vi "Compensator.vi"() -> ()   [LabVIEW 2010]
uses:
  <vilib>/Platform/TimedLoop/XDataNode/XDataNode.xnode
  <vilib>/Platform/TimedLoop/XDataNode/timing_clust.ctl
  <vilib>/Platform/TimedLoop/XDataNode/nitl_modes.ctl
  <vilib>/Platform/TimedLoop/XDataNode/wakeup.ctl
  <vilib>/Platform/TimedLoop/XDataNode/XDNodeRunTimeDep.lvlib
panel:
  out "data":dbl
  out "Finished Late?":bool
  out "XY Graph":cluster{"Y":dbl[], "Y":dbl[]}[](graph)
  in  "Analyze":bool
  in  "Frequency (Hz)":dbl
  in  "Amplitude":dbl
  in  "DC Offset":dbl
  in  "Phase (Degrees)":dbl
  out "Waveform Chart":dynamicdata(graph)
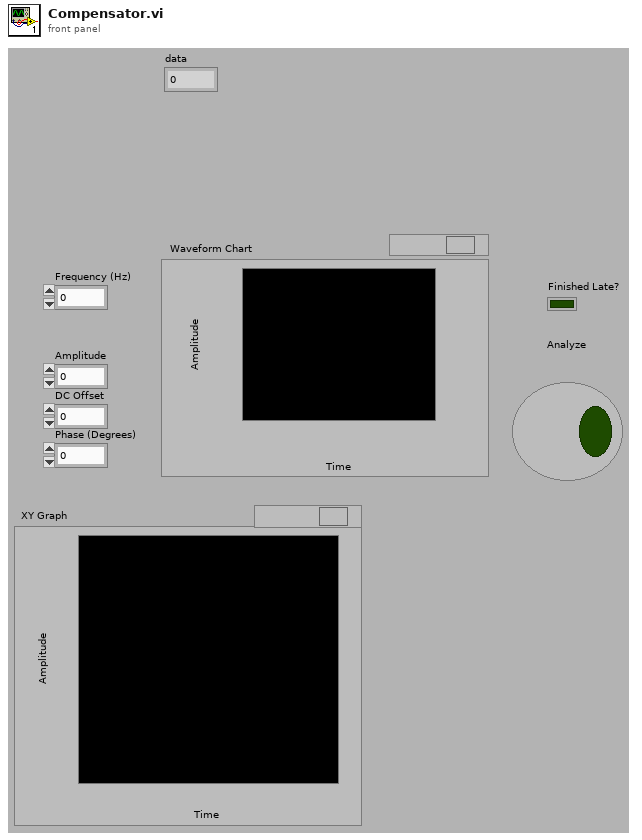
[diagram p1: front panel]
types:
  T1 = typedef "XDNodeRunTimeDep.lvlib/timing_clust.ctl" = cluster{"Expected End [f-1]":u64, "Actual End [f-1]":u64, "Finished Late? [f-1]":bool, "Expected End [i-1]":u64, "Actual End [i-1]":u64, "Finished Late? [i-1]":bool, "Expected Start [i]":u64, "Actual Start [i]":u64, "Expected Start [f]":u64, "Actual Start [f]":u64, "Source Name":string, "Structure Name":string, "Period":i64, "Deadline":i64, "Offset":i64, "Start":i64, "Priority":i32, "Timeout":i32, "Mode":T2, "Wakeup Reason":T3, "Error":errorcluster, "Source Type":string, "Secondary Source Type":string, "Global End Time":u64, "Global Start Time":u64, "Frame Duration":u64, "Iteration Duration":u64, "Assigned CPU":i32, "I/O Scan Engine Mode":u32}
  T2 = typedef "XDNodeRunTimeDep.lvlib/nitl_modes.ctl" = enum32{"No Change", "Process missed periods, maintain original phase", "Discard missed periods, maintain original phase", "Process missed periods, ignore original phase", "Discard missed periods, ignore original phase"}
  T3 = typedef "XDNodeRunTimeDep.lvlib/wakeup.ctl" = enum32{"Normal", "Aborted", "Asynchronous wakeup", "Timing source error", "Timed loop error", "Timeout"}
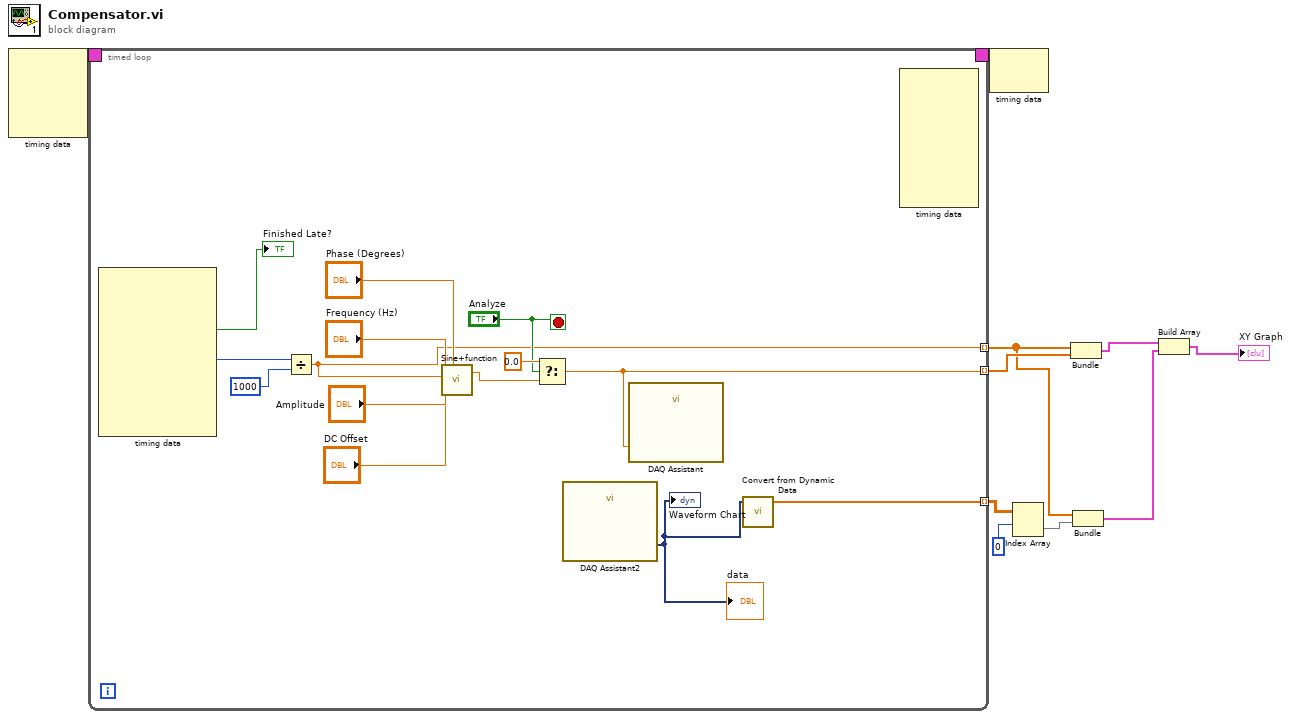
[diagram p0: block diagram]
diagram:
  n1 = node-c288() -> (w10:T1)  [unwired: 4 in]
  n2 = timed-loop {
    timing: w10 -> [_]
    timing-out: [_] -> w9
    tunnel: [w15] -> w8 mode=indexing
    tunnel: [w13] -> w7 mode=indexing
    tunnel: [w12] -> w4 mode=indexing
    stop <- "Analyze" stop-if-true
    n3 = node-c288() -> (→"Finished Late?":bool, w20:i64)  [unwired: 1 in, 8 out]
    n4 = Divide(x=w20, y=1000) -> (x/y=w12:dbl)
    n5 = call "Sine+function.vi"("Frequency (Hz)"="Frequency (Hz)", "Time (Sec)"=w12, "Amplitude"="Amplitude", "DC Offset"="DC Offset", "Phase (Degrees)"="Phase (Degrees)") -> ("A*sin(2*pi*f*t+phi)+B"=w18:dbl)  [unwired: 1 in]
    n6 = Select(t=0.0, s="Analyze", f=w18) -> (s? t:f=w15:dbl)
    n7 = call "DAQ Assistant2"() -> ("data"=w14:dynamicdata)  [unwired: 17 in, 2 out]
    "Waveform Chart" <- w14
    "data" <- w14
    n8 = call "DAQ Assistant"("data"=w15) -> ()  [unwired: 17 in, 2 out]
    n9 = call "Convert from Dynamic Data"("Dynamic Data Type"=w14) -> ("Array"=w13:dbl[])  [unwired: 3 in]
    n10 = node-c288() -> ()  [unwired: 8 in, 1 out]
  }
  n11 = node-c288(w9) -> ()  [unwired: 1 out]
  n12 = Index Array(array=w7, index (row)=0 ("index")) -> (element=w5:dbl[])  [unwired: 1 in]
  n13 = Bundle(w4, w8) -> (w2:cluster{dbl[], dbl[]})  [unwired: 1 in]
  n14 = Bundle(w4, "Array"=w5) -> (w1:cluster{dbl[], "Array":dbl[]})  [unwired: 1 in]
  n15 = Build Array(w2, w1) -> (→"XY Graph":cluster{dbl[], "Array":dbl[]}[])
